vi "GA Open.vi"(8 "error in (no error)":errorcluster caption="错误输入（无错误）", 10 "cName":string, 11 "iType":i16) -> (0 "error out":errorcluster caption="错误输出", 2 "cName out":string, 3 "function return":i32)   [LabVIEW 2024, in "GAS.lvlib"]
doc: "extern \"C\" __declspec(dllimport) int GA_Open(short iType=0,char* cName=\"COM1\");"
uses:
  GAS.lvlib
  GAS.dll
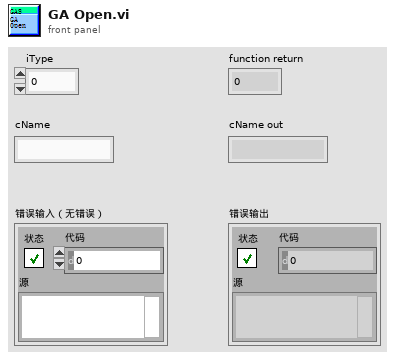
[diagram p1: front panel]
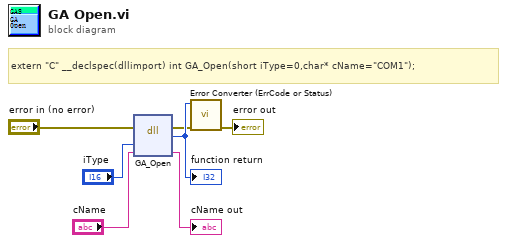
[diagram p0: block diagram]
diagram:
  # "extern \"C\" __declspec(dllimport) int GA_Open(short iType=0,char* cName=\"COM1\");"
  n1 = dll-call lib="PTH2?abs D实验室软件（勿删）集成测试系统GAS.*" fn="GA_Open"(error in="error in (no error)", "iType"="iType", "cName"="cName") -> (error out=w2:errorcluster, w7:i32, "cName"=→"cName out":string)  [unwired: 3 in, 1 out]
  "function return" <- w7
  n2 = call "Error Converter (ErrCode or Status).vi"("error in (no error)"=w2, "error code"=w7) -> ("error out"=→"error out":errorcluster)  [unwired: 9 in]
